vi "Four Track - Main.vi"() -> ()   [LabVIEW 2014]
uses:
  Sub VIs/Audio/Controls/Delay Controls.ctl
  File Controls.ctl
  Playback Controls.ctl
  Track Controls.ctl
  Track Settings.ctl
  Track Effects Settings.ctl
  Track Volume Settings.ctl
  Sub VIs/Audio/Controls/playback state.ctl
  Audio In.ctl
  <vilib>/FPGAPlugInAG/myRIO-1900/niLvFpga_Open_myRIO-1900.vi
  <vilib>/rvi/interface/common/dynamic/niFpgaDynamicAddResources.vi
  Sub VIs/Audio/Controls/sample block size.vi
  <vilib>/FPGAPlugInAG/Dynamic/niLvFpga_Close_Dynamic.vi
  <vilib>/rvi/interface/nirviOpenFPGA/nirviOpenFPGA.xnode
  FPGA Bitfiles/mySynth_FPGATarget_FPGAMain_WASpsvx+XwM.lvbitx
  FPGA Main.vi
  <vilib>/rvi/interface/nirviCloseFPGA/nirviCloseFPGA.xnode
panel:
  in  "Measures":i32
  in  "BPM":i32
  in  "Time Signature":enum16{"4/4", "3/4"}(ring)
  out "Right":i16[](graph)
  out "Left":i16[](graph)
  in  "stop":bool
  out "Playback State":T1
  out "error out":errorcluster
  in  "Track Controls":T2={"Track 0"={"Effects Settings"={"Delay"=4.86522497566e-313, "Delay 2"=4.86522497566e-313}, "Volume Settings"={"Mute"=FALSE, "Solo"=FALSE, "Record"=FALSE, "Pan"=4.86522497566e-313, "Volume"=4.86522497566e-313}}, "Track 1"={"Effects Settings"={"Delay"=0.0, "Delay 2"=0.0}, "Volume Settings"={"Mute"=FALSE, "Solo"=FALSE, "Record"=FALSE, "Pan"=0.0, "Volume"=0.0}}, "Track 2"={"Effects Settings"={"Delay"=0.0, "Delay 2"=0.0}, "Volume Settings"={"Mute"=FALSE, "Solo"=FALSE, "Record"=FALSE, "Pan"=0.0, "Volume"=0.0}}, "Track 3"={"Effects Settings"={"Delay"=0.0, "Delay 2"=0.0}, "Volume Settings"={"Mute"=FALSE, "Solo"=FALSE, "Record"=FALSE, "Pan"=0.0, "Volume"=0.0}}} {"Track 3"."Volume Settings"."Volume" scale=1.0..10.0; "Track 3"."Volume Settings"."Pan" scale=0.0..1.0; "Track 3"."Effects Settings"."Delay 2" scale=0.0..10.0; "Track 3"."Effects Settings"."Delay" scale=0.0..1.0; "Track 2"."Volume Settings"."Volume" scale=1.0..10.0; "Track 2"."Volume Settings"."Pan" scale=0.0..1.0; "Track 2"."Effects Settings"."Delay 2" scale=0.0..10.0; "Track 2"."Effects Settings"."Delay" scale=0.0..1.0; "Track 1"."Volume Settings"."Volume" scale=1.0..10.0; "Track 1"."Volume Settings"."Pan" scale=0.0..1.0; "Track 1"."Effects Settings"."Delay 2" scale=0.0..10.0; "Track 1"."Effects Settings"."Delay" scale=0.0..1.0; "Track 0"."Volume Settings"."Volume" scale=1.0..10.0; "Track 0"."Volume Settings"."Pan" scale=0.0..1.0; "Track 0"."Effects Settings"."Delay 2" scale=0.0..10.0; "Track 0"."Effects Settings"."Delay" scale=0.0..1.0}
  in  "Playback Controls":T6
  in  "File Controls":T7
  in  "Delay Settings":T8 {"Wet/Dry" scale=0.0..5.0}
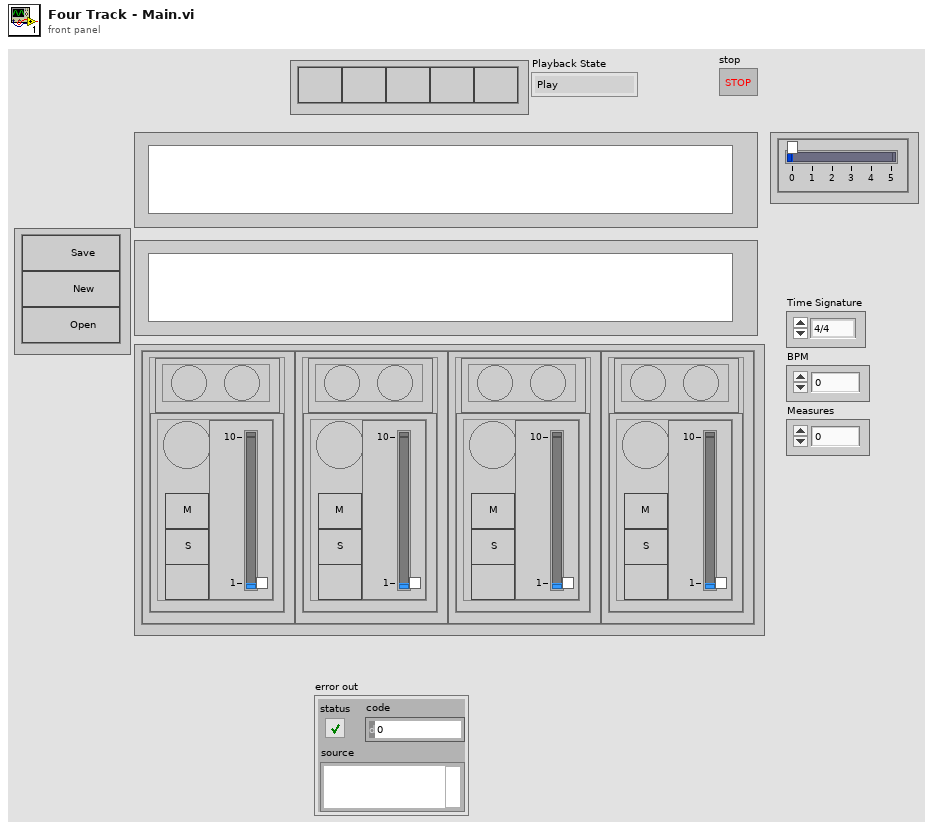
[diagram p1: front panel]
types:
  T1 = typedef "playback state.ctl" = enum16{"Play", "Record", "Stop", "Pause", "Rewind"}
  T2 = typedef "Track Controls.ctl" = cluster{"Track 0":T3, "Track 1":T3, "Track 2":T3, "Track 3":T3}
  T3 = typedef "Track Settings.ctl" = cluster{"Effects Settings":T4, "Volume Settings":T5}
  T4 = typedef "Track Effects Settings.ctl" = cluster{"Delay":dbl, "Delay 2":dbl}
  T5 = typedef "Track Volume Settings.ctl" = cluster{"Mute":bool, "Solo":bool, "Record":bool, "Pan":dbl, "Volume":dbl}
  T6 = typedef "Playback Controls.ctl" = cluster{"Play Button":bool, "Record Button":bool, "Media Stop Button":bool, "Pause Button":bool, "Skip Back Button":bool}
  T7 = typedef "File Controls.ctl" = cluster{"Save Button":bool, "New Button":bool, "Open Button":bool}
  T8 = typedef "Delay Controls.ctl" = cluster{"Wet/Dry":u8}
  T9 = typedef "Track (File) References.ctl" = cluster{"Track_1_Ref":refnum<k34>, "Track_2_Ref":refnum<k34>, "Track_3_Ref":refnum<k34>, "Track_4_Ref":refnum<k34>, "Track_Name_1":string, "Track_Name_2":string, "Track_Name_3":string, "Track_Name_4":string}
  T10 = typedef "Audio In.ctl" = cluster{"AudioIn/Left (N Samples)":i16[], "AudioIn/Right (N Samples)":i16[]}
  T11 = typedef "4 Track Audio.ctl" = cluster{"Track 0":T10, "Track 1":T10, "Track 2":T10, "Track 3":T10}
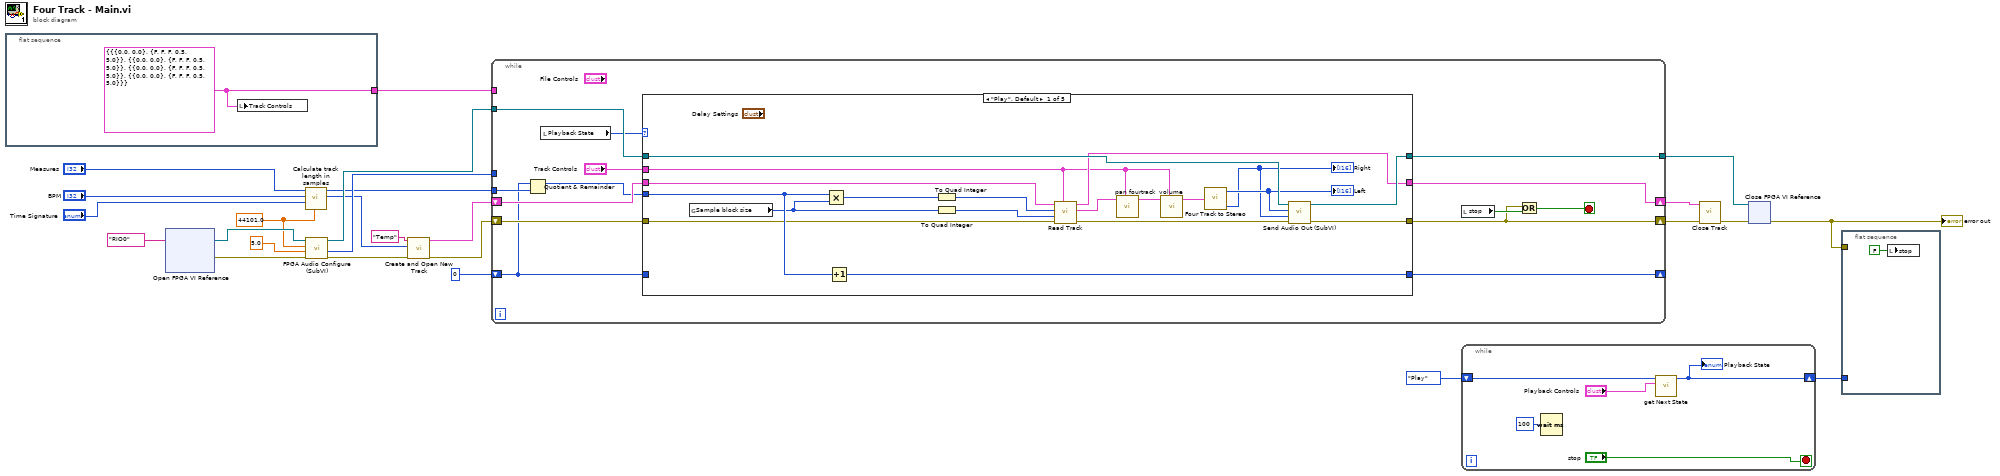
[diagram p0: block diagram]
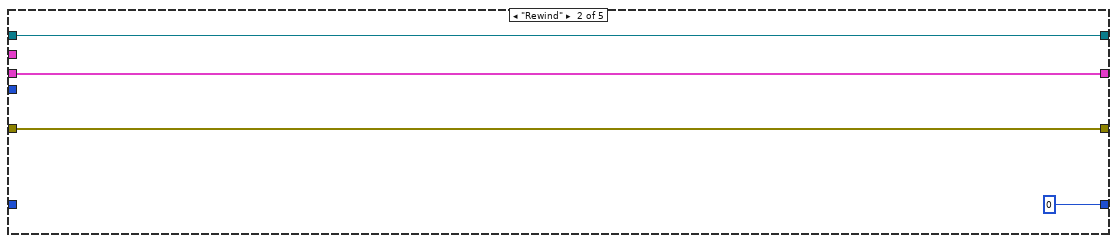
[diagram p2: hidden frame]
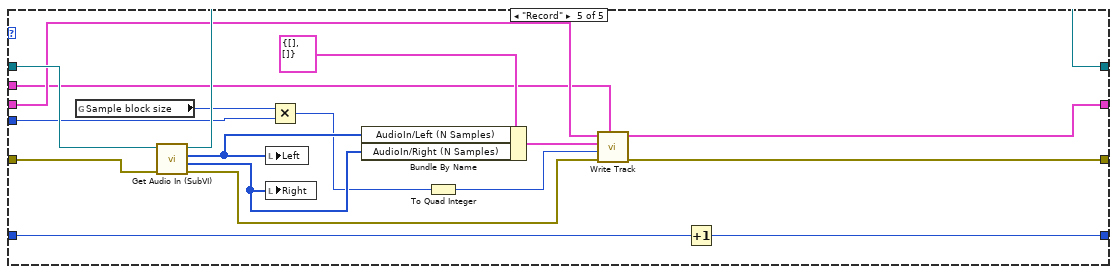
[diagram p5: hidden frame]
diagram:
  w6 = 44101.0 ("Sample Rate (Hz)")
  n1 = flat-sequence {
    tunnel: [w26] -> w22
    frame #0 {
      w26 = T2 {"Track 0"={"Effects Settings"={"Delay"=0.0, "Delay 2"=0.0}, "Volume Settings"={"Mute"=FALSE, "Solo"=FALSE, "Record"=FALSE, "Pan"=0.5, "Volume"=5.0}}, "Track 1"={"Effects Settings"={"Delay"=0.0, "Delay 2"=0.0}, "Volume Settings"={"Mute"=FALSE, "Solo"=FALSE, "Record"=FALSE, "Pan"=0.5, "Volume"=5.0}}, "Track 2"={"Effects Settings"={"Delay"=0.0, "Delay 2"=0.0}, "Volume Settings"={"Mute"=FALSE, "Solo"=FALSE, "Record"=FALSE, "Pan"=0.5, "Volume"=5.0}}, "Track 3"={"Effects Settings"={"Delay"=0.0, "Delay 2"=0.0}, "Volume Settings"={"Mute"=FALSE, "Solo"=FALSE, "Record"=FALSE, "Pan"=0.5, "Volume"=5.0}}} ("Track Controls 2")
      n2 = local write "Track Controls"(w26) -> ()
    }
  }
  n3 = xnode "Open FPGA VI Reference"("resource name"=tag "RIO0") -> ("FPGA VI Reference Out"=w17:refnum<k20>, "error out"=w16:errorcluster)  [unwired: 1 in]
  n4 = call "Calculate track length in samples.vi"("Sample Rate (Hz)"=w6, "Time Signature"="Time Signature", "BPM"="BPM", "Measures"="Measures") -> ("Track Length in Samples"=w2:i32, "Track Division in Samples"=w1:i32)  [unwired: 6 in]
  n5 = call "FPGA Audio Configure (SubVI).vi"("error in (no error)"=w16, "Read Rate (Hz)"=5.0, "Audio Sample Rate (Hz)"=w6, "Refnum in"=w17) -> ("error out"=w8:errorcluster, "Required loop period (ms)"=w20:u32, "Refnum out"=w21:refnum<k20>)  [unwired: 4 in, 1 out]
  n6 = call "Create and Open New Track.vi"("Error In"=w8, "Samples Per Channel"=w2, "Track Name"="Temp") -> ("Error Out"=w7:errorcluster, "Track (File) References"=w12:T9)  [unwired: 7 in]
  n7 = while {
    shift-right: [w30] -> w11
    shift-left: w12 -> [w31]
    shift-right: [w35] -> w10
    shift-left: w7 -> [w38]
    shift-right: [w33] -> _
    shift-left: 0 -> [w27]
    tunnel: w22 -> [_]
    tunnel: w21 -> [w39]
    tunnel: [w32] -> w15
    tunnel: w20 -> [_]
    tunnel: w1 -> [w29]
    stop <- w34 stop-if-true
    n8 = Quotient & Remainder(x=w27, y=w29) -> (x-y*floor(x/y)=w28:i32)  [unwired: 1 out]
    n9 = local read "Playback State"() -> (w37:T1)
    n10 = case shown="\"Play\", Default" w37 {
      tunnel: "Track Controls" -> [w41 _ _ _ w73]
      tunnel: w39 -> [w57 w61 w65 w69 w88]
      tunnel: w38 -> [w48 w63 w67 w71 w87]
      tunnel: [w56 w63 w67 w71 w80] -> w35
      tunnel: w28 -> [w52 _ w66 w70 w79]
      tunnel: [w59 0 w66 w70 w89] -> w33
      tunnel: [w55 w61 w65 w69 w86] -> w32
      tunnel: w31 -> [w51 w60 w64 w68 w85]
      tunnel: [w50 w60 w64 w68 w84] -> w30
      tunnel: w27 -> [_ _ _ _ w72]
      frame "Play", Default {
        n11 = global read "sample block size.vi" "Sample block size"() -> (w42:i32)
        n12 = Multiply(x=w52, y=w42) -> (x*y=w45:i32)
        n13 = Increment(x=w52) -> (x+1=w59:i32)
        n14 = To Quad Integer(1:w45) -> (0:w44:i64)
        n15 = To Quad Integer(1:w42) -> (0:w43:i64)
        n16 = call "Read Track.vi"("Track Controls"=w41, "Error In"=w48, "Number Of Elements to Read"=w43, "Read Position"=w44, "Track (File) References In"=w51) -> ("Error Out"=w47:errorcluster, "4-Track Audio"=w49:T11, "Track (File) References Out"=w50:T9)  [unwired: 4 in]
        n17 = call "pan fourtrack.vi"("Track Controls"=w41, "4-Track Audio in"=w49) -> ("4-Track Audio out"=w58:T11)  [unwired: 9 in]
        n18 = call "volume.vi"("Track Controls"=w41, "4-Track Audio in"=w58) -> ("4-Track Audio out"=w46:T11)  [unwired: 9 in]
        n19 = call "Four Track to Stereo.vi"("4-Track Audio In"=w46) -> ("Right Out"=w53:i16[], "Left Out"=w54:i16[])  [unwired: 3 in]
        "Left" <- w54
        "Right" <- w53
        n20 = call "Send Audio Out (SubVI).vi"("error in (no error)"=w47, "Right Audio Out"=w53, "Left Audio Out"=w54, "Refnum in"=w57) -> ("error out"=w56:errorcluster, "Refnum out"=w55:refnum<k20>)  [unwired: 6 in]
      }
      frame "Rewind" {
      }
      frame "Stop" {
      }
      frame "Pause" {
      }
      frame "Record" {
        n21 = global read "sample block size.vi" "Sample block size"() -> (w77:i32)
        n22 = call "Get Audio In (SubVI).vi"("error in (no error)"=w87, "Refnum in"=w88) -> ("error out"=w81:errorcluster, "Right Audio In"=w76:i16[], "Left Audio In"=w78:i16[], "Refnum out"=w86:refnum<k20>)  [unwired: 6 in]
        n23 = local write "Left"(w78) -> ()
        n24 = local write "Right"(w76) -> ()
        n25 = Multiply(x=w77, y=w79) -> (x*y=w74:i32)
        n26 = Bundle By Name(cluster=T10 {"AudioIn/Left (N Samples)"=[], "AudioIn/Right (N Samples)"=[]} ("Audio In"), "AudioIn/Left (N Samples)"=w78, "AudioIn/Right (N Samples)"=w76) -> (w82:T10)
        n27 = To Quad Integer(1:w74) -> (0:w75:i64)
        n28 = call "Write Track.vi"("Track Controls"=w73, "Error In"=w81, "Write Position"=w75, "Audio In"=w82, "Track (File) References In"=w85) -> ("Error Out"=w80:errorcluster, "Track (File) References Out"=w84:T9)  [unwired: 5 in]
        n29 = Increment(x=w72) -> (x+1=w89:i32)
      }
    }
    n30 = local read "stop"() -> (w36:bool)
    n31 = Or(x=w35, y=w36) -> (x .or. y?=w34:bool)
  }
  n32 = while {
    shift-right: [w91] -> w24
    shift-left: playback_state."Play" ("Playback State") -> [w90]
    stop <- "stop" stop-if-true
    n33 = Wait (ms)(milliseconds to wait=u32 100) -> ()  [unwired: 1 out]
    n34 = call "get Next State.vi"("Playback Controls"="Playback Controls", "Playback State in"=w90) -> ("Playback State out"=w91:T1)  [unwired: 9 in]
    "Playback State" <- w91
  }
  n35 = call "Close Track.vi"("Error In"=w10, "Track (File) References"=w11) -> ("Error Out"=w9:errorcluster)  [unwired: 9 in]
  n36 = xnode "Close FPGA VI Reference"("FPGA VI Reference In"=w15, "error in"=w9) -> ("error out"=w14:errorcluster)
  "error out" <- w14
  n37 = flat-sequence {
    tunnel: w14 -> [_]
    tunnel: w24 -> [_]
    frame #0 {
      n38 = local write "stop"(FALSE ("stop")) -> ()
    }
  }
